vi "get IP Address.vi"(8 "error in (no error)":errorcluster) -> (0 "error out":errorcluster, 2 "IP Address":string[](array[string]))   [LabVIEW 2020]
panel:
  out "name":string
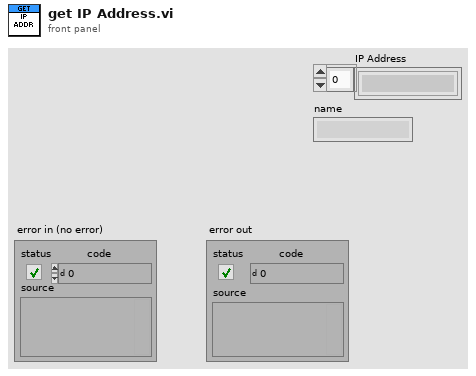
[diagram p1: front panel]
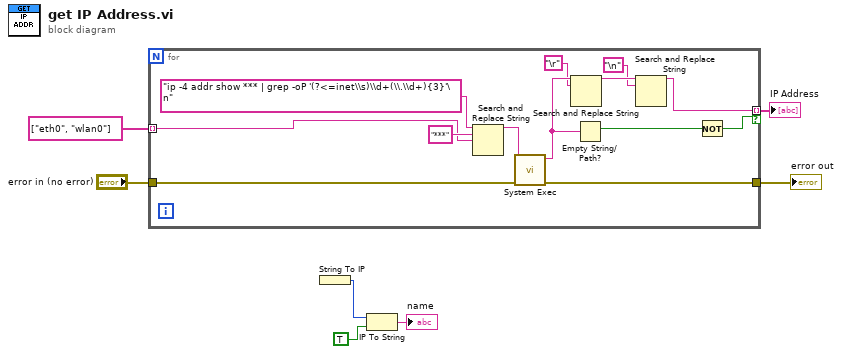
[diagram p0: block diagram]
diagram:
  n1 = for {
    tunnel: string[] ["eth0", "wlan0"] -> [w17] mode=indexing
    tunnel: [w8] -> w6 mode=indexing if=w15
    tunnel: "error in (no error)" -> [w13]
    tunnel: [w14] -> w4
    n2 = Search and Replace String(input string="ip -4 addr show *** | grep -oP '(?<=inet\\s)\\d+(\\.\\d+){3}'\n" ("command line"), search string="***", replace string=w17) -> (result string=w20:string)  [unwired: 5 in, 3 out]
    n3 = call <vilib>:"System Exec.vi"("error in (no error)"=w13, "command line"=w20) -> ("error out"=w14:errorcluster, "standard output"=w12:string)  [unwired: 6 in, 2 out]
    n4 = Search and Replace String(input string=w12, search string="\r") -> (result string=w10:string)  [unwired: 6 in, 3 out]
    n5 = Empty String/Path?(string/path=w12) -> (empty?=w16:bool)
    n6 = Search and Replace String(input string=w10, search string="\n") -> (result string=w8:string)  [unwired: 6 in, 3 out]
    n7 = Not(x=w16) -> (.not. x?=w15:bool)
  }
  "IP Address" <- w6
  "error out" <- w4
  n8 = String To IP() -> (0:w2:u32)  [unwired: 1 in]
  n9 = IP To String(1:TRUE ("dot notation? (F)"), 2:w2) -> (0:→"name":string)
